vi "Write Host Name.vi"(8 "error in (no error)":errorcluster, 10 "Host Name":string, 11 "Board in":refnum<class "Board.lvclass">) -> (0 "error out":errorcluster, 3 "Board out":refnum<class "Board.lvclass">)   [LabVIEW 2025, in "SW License Manager.lvlib" / "Board.lvclass"]
uses:
  Board.lvclass
  Board.lvclass/Board.ctl
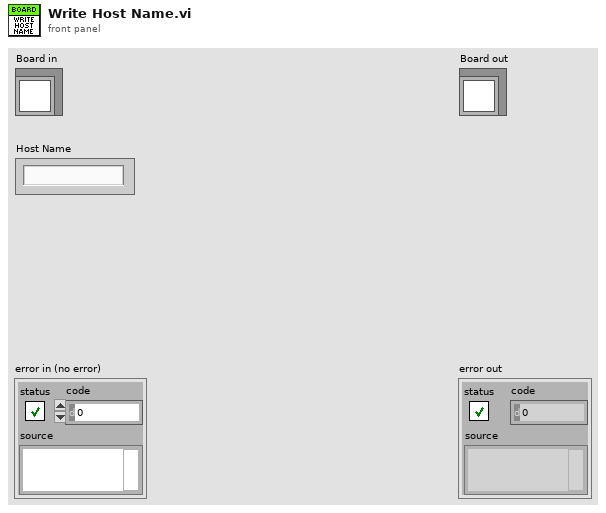
[diagram p1: front panel]
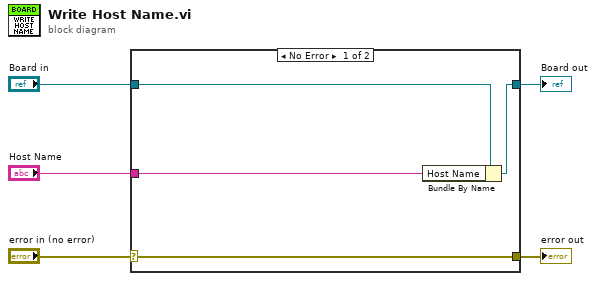
[diagram p0: block diagram]
diagram:
  n1 = case shown="No Error" "error in (no error)" {
    selector: "error in (no error)" -> [w9 w10]
    tunnel: [w9 w10] -> w4
    tunnel: [w7 w11] -> w2
    tunnel: "Board in" -> [w8 w11]
    tunnel: "Host Name" -> [w6 _]
    frame No Error {
      n2 = Bundle By Name(cluster=w8, "Host Name"=w6) -> (w7:refnum<class "Board.lvclass">)
    }
    frame Error {
    }
  }
  "error out" <- w4
  "Board out" <- w2
